vi "Dresser DXD Initialize.vi"(0 "Serial Port (COM1)":refnum<visa-resource-name>="COM1", 1 "DXD Address (1)":T1=1 min=1 max=99 step=1, 2 "Serial Stop Bits (1)":u16(ring)=10 items=["1.0"=10, "1.5"=15, "2.0"=20], 3 "Termination Character (T, <lf>)":bool=TRUE caption="<lf>\n<cr>", 5 "error in (no error)":errorcluster, 6 "Serial Parity (even)":u16(ring)=2 items=["None", "Odd", "Even", "Mark", "Space"], 7 "ID Query (T: Check)":bool=TRUE, 8 "Serial Flow Control (None)":u16(ring) items=["None"=0, "XON/XOFF"=1, "RTS/CTS"=2, "DTR/DSR"=4], 10 "Serial Data Bits (7)":u16=7, 11 "Reset (F: Don't Reset)":bool, 12 "Serial Baud Rate (19200)":u16(ring)=4 items=["1200", "2400", "4800", "9600", "19200", "38400", "57600", "115200"]) -> (14 "VISA session":refnum<visa-resource-name>, 15 "Returned String":string, 19 "Error Out":errorcluster)   [LabVIEW 2015]
doc: "This VI is used to establish communication with a Dresser DXD Series pressure transducer. The function has an instrument descriptor string as an input. Also, the VI can perform user selectable ID query and/or reset operations.\n\nThis VI passes the addressing information in the instrument descriptor to the VISA Open VI and returns the Dresser DXD Series pressure transducer ID. You must run this VI before using any of the data, utility, or application example VIs for this device.\n\nWritten by:\nBLOOMY CONTROLS, INC\nWINDSOR, CT 06095, USA\n860-298-9925\nwww.bloomy.com\nV2.0.0\nMay, 2002"
uses:
  Type Defs/DXD Address.ctl
panel:
  # "For instructions on the use of this VI, press Ctrl+H to display the help window and move the mouse over the icon, controls, and indicators"
  # "Check\n\n\nDon't Check"
  # "Reset (!CAUTION!)\n\nDon't Reset"
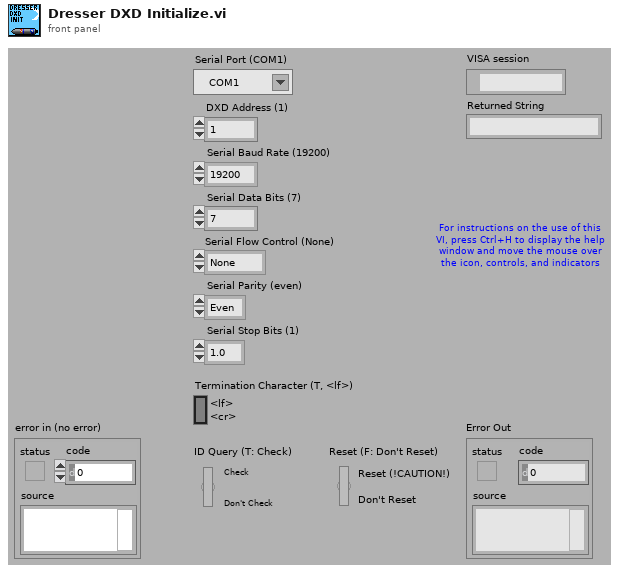
[diagram p1: front panel]
types:
  T1 = typedef "DXD Address.ctl" = i32
  T2 = cluster{"status":bool, "code":i32, "VI Name":string}
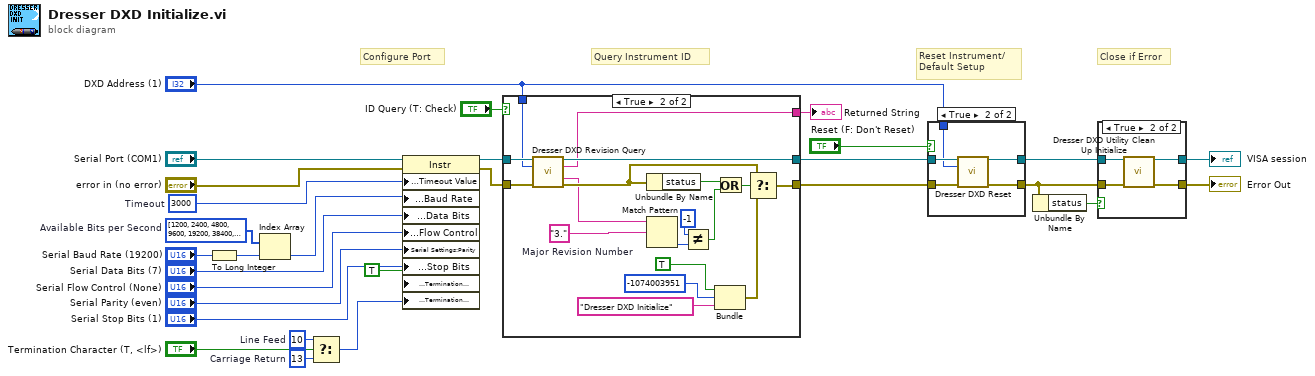
[diagram p0: block diagram]
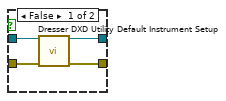
[diagram p3: hidden frame]
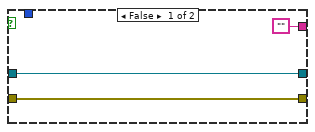
[diagram p4: hidden frame]
diagram:
  w4 = u8 10  # Line Feed
  w3 = u8 13  # Carriage Return
  w18 = u32[] [1200, 2400, 4800, 9600, 19200, 38400, 57600, 115200]  # Available Bits per Second
  w20 = u32 3000  # Timeout
  # "Close if Error"
  # "Query Instrument ID"
  # "Reset Instrument/\nDefault Setup"
  # "Configure Port"
  n1 = To Long Integer(number="Serial Baud Rate (19200)") -> (32bit integer=w12:i32)
  n2 = Index Array(array=w18, index=w12) -> (element=w19:u32)
  n3 = Select(t=w4, s="Termination Character (T, <lf>)", f=w3) -> (s? t:f=w1:u8)
  n4 = property class="Instr"(reference="Serial Port (COM1)", error in="error in (no error)", "General Settings:Timeout Value"=w20, "Serial Settings:Baud Rate"=w19, "Serial Settings:Data Bits"="Serial Data Bits (7)", "Serial Settings:Flow Control"="Serial Flow Control (None)", "Serial Settings:Parity"="Serial Parity (even)", "Serial Settings:Stop Bits"="Serial Stop Bits (1)", "Message Based Settings:Termination Character Enable"=TRUE, "Message Based Settings:Termination Character"=w1) -> (reference out=w11:refnum<visa-resource-name>, error out=w10:errorcluster)
  n5 = case shown="True" "ID Query (T: Check)" {
    tunnel: [w31 w50] -> w28
    tunnel: [w32 w37] -> w29
    tunnel: w11 -> [w32 w40]
    tunnel: w10 -> [w31 w39]
    tunnel: "DXD Address (1)" -> [_ w38]
    tunnel: ["" w33] -> w6
    frame False {
    }
    frame True {
      w34 = "3."  # Major Revision Number
      n6 = call "Dresser DXD Revision Query.vi"("VISA session"=w40, "Device Address (1)"=w38, "Error In (no error)"=w39) -> ("dup VISA session"=w37:refnum<visa-resource-name>, "Returned String"=w33:string, "Instr Firmware Revision"=w35:string, "Error Out"=w36:errorcluster)  [unwired: 8 in, 1 out]
      n7 = Unbundle By Name(w36) -> ("status"=w46:bool)
      n8 = Match Pattern(string=w35, regular expression=w34) -> (offset past match=w44:i32)  [unwired: 1 in, 3 out]
      n9 = Not Equal?(x=-1, y=w44) -> (x != y?=w48:bool)
      n10 = Bundle(TRUE, -1074003951, "VI Name"="Dresser DXD Initialize") -> (w43:cluster{bool, i32, "VI Name":string})  [unwired: 1 in]
      n11 = Or(x=w46, y=w48) -> (x .or. y?=w47:bool)
      n12 = Select(t=w36, s=w47, f=w43) -> (s? t:f=w50:T2)
    }
  }
  "Returned String" <- w6
  n13 = case shown="True" "Reset (F: Don't Reset)" {
    tunnel: w28 -> [w53 w56]
    tunnel: [w52 w59] -> w24
    tunnel: w29 -> [w54 w57]
    tunnel: [w51 w58] -> w23
    tunnel: "DXD Address (1)" -> [_ w55]
    frame False {
      n14 = call "Dresser DXD Utility Default Instrument Setup.vi"("VISA session"=w54, "Error In (no error)"=w53) -> ("dup VISA session"=w51:refnum<visa-resource-name>, "Error Out"=w52:errorcluster)  [unwired: 12 in]
    }
    frame True {
      n15 = call "Dresser DXD Reset.vi"("VISA session"=w57, "DXD Address (1)"=w55, "Error In (no error)"=w56) -> ("dup VISA session"=w58:refnum<visa-resource-name>, "Error Out"=w59:errorcluster)  [unwired: 11 in]
    }
  }
  n16 = Unbundle By Name(w24) -> ("status"=w25:bool)
  n17 = case shown="True" w25 {
    tunnel: w23 -> [w61 w65]
    tunnel: w24 -> [w60 w64]
    tunnel: [w61 w63] -> w22
    tunnel: [w60 w62] -> w21
    frame False {
    }
    frame True {
      n18 = call "Dresser DXD Utility Clean Up Initialize.vi"("VISA session"=w65, "Error In (no error)"=w64) -> ("dup VISA session"=w63:refnum<visa-resource-name>, "Error Out"=w62:errorcluster)  [unwired: 12 in]
    }
  }
  "VISA session" <- w22
  "Error Out" <- w21
